vi "login.vi"(8 "error in":errorcluster) -> (0 "error out":errorcluster, 2 "Headers":string[](array[string]))   [LabVIEW 2022 SP3]
uses:
  <vilib>/Utility/SMTP/NI_SMTPEmail.lvlib
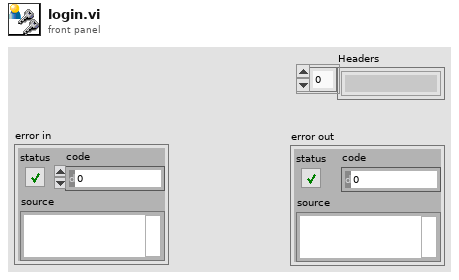
[diagram p1: front panel]
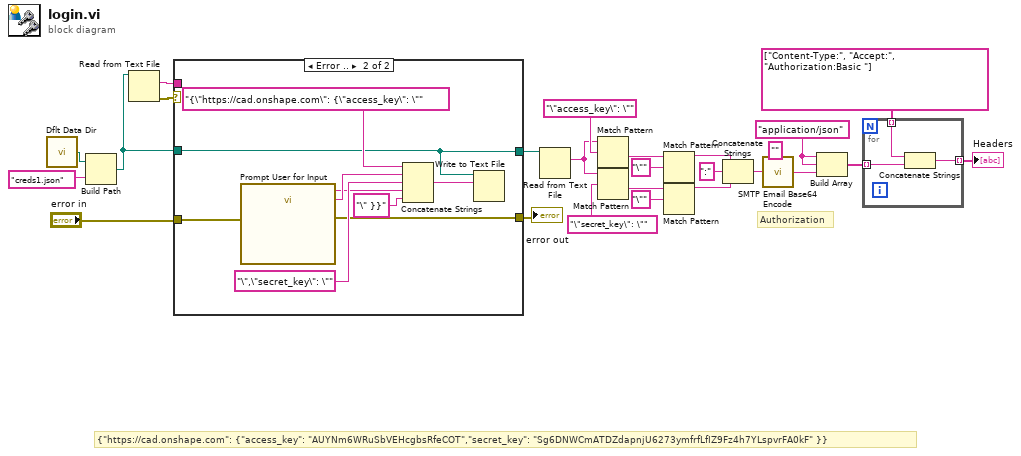
[diagram p0: block diagram]
diagram:
  w4 = "application/json"
  # "{\"https://cad.onshape.com\": {\"access_key\": \"AUYNm6WRuSbVEHcgbsRfeCOT\",\"secret_key\": \"Sg6DNWCmATDZdapnjU6273ymfrfLfIZ9Fz4h7YLspvrFA0kF\" }}"
  # "Authorization"
  n1 = call <vilib>:"Dflt Data Dir.vi"() -> ("App:Default Data Directory"=w17:path)
  n2 = Build Path(base path=w17, name or relative path="creds1.json") -> (appended path=w15:path)
  n3 = Read from Text File(file (use dialog)=w15) -> (text=w24:string, error out=w25:errorcluster)  [unwired: 3 in, 2 out]
  n4 = case shown="Error .." w25 {
    tunnel: w24 -> [_ _]
    tunnel: w15 -> [w26 w29]
    tunnel: [w26 w29] -> w14
    tunnel: "error in" -> [_ w28]
    tunnel: [_ w27] -> w12
    frame No Error {
    }
    frame Error {
      n5 = call "Prompt User for Input"("error in (no error)"=w28) -> ("secret_key"=w32:string, "access_key"=w34:string, "error out"=w27:errorcluster)  [unwired: 15 in, 1 out]
      n6 = Concatenate Strings("{\"https://cad.onshape.com\": {\"access_key\": \"", w34, "\",\"secret_key\": \"", w32, "\" }}") -> (w30:string)
      n7 = Write to Text File(file (use dialog)=w29, text=w30) -> ()  [unwired: 2 in, 3 out]
    }
  }
  "error out" <- w12
  n8 = Read from Text File(file (use dialog)=w14) -> (text=w11:string)  [unwired: 3 in, 3 out]
  n9 = Match Pattern(string=w11, regular expression="\"access_key\": \"") -> (after substring=w22:string)  [unwired: 1 in, 3 out]
  n10 = Match Pattern(string=w11, regular expression="\"secret_key\": \"") -> (after substring=w23:string)  [unwired: 1 in, 3 out]
  n11 = Match Pattern(string=w22, regular expression="\"") -> (before substring=w3:string)  [unwired: 1 in, 3 out]
  n12 = Match Pattern(string=w23, regular expression="\"") -> (before substring=w2:string)  [unwired: 1 in, 3 out]
  n13 = Concatenate Strings(w3, ":" ("string"), w2) -> (w7:string)
  n14 = call <vilib>:"SMTP Email Base64 Encode.vi"("Normal String"=w7, "Line separator (\\n)"="" ("Line separator (\\n)")) -> ("Base64 String"=w5:string)
  n15 = Build Array(w4, w4, w5) -> (w9:string[])
  n16 = for {
    tunnel: string[] ["Content-Type:", "Accept:", "Authorization:Basic "] -> [w38] mode=indexing
    tunnel: w9 -> [w37] mode=indexing
    tunnel: [w36] -> w1 mode=indexing
    n17 = Concatenate Strings(w38, w37) -> (w36:string)
  }
  "Headers" <- w1
